vi "Create Default Attributes.vi"(5 "Unique ID":string, 7 "Process Executive Ref":refnum<data-value>, 11 "Wait in":refnum<class "Wait.lvclass">) -> (3 "Wait out":refnum<class "Wait.lvclass">)   [LabVIEW 2019, in "Wait.lvclass"]
uses:
  <vilib>/gpm_packages/@cs/Car-wash/Source/Process Steps/Wait/Wait.lvclass
  <vilib>/gpm_packages/@cs/test-executive/Source/Test Executive/ITestExecutive/ITest Executive.lvclass
  3f0b96d9-ec26-4894-9d74-60fba4d816d8.vi
  <vilib>/Utility/error.llb/Error Cluster From Error Code.vi
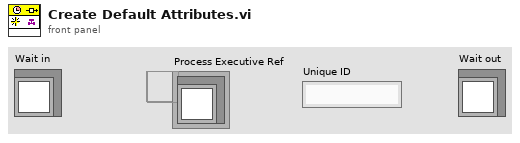
[diagram p1: front panel]
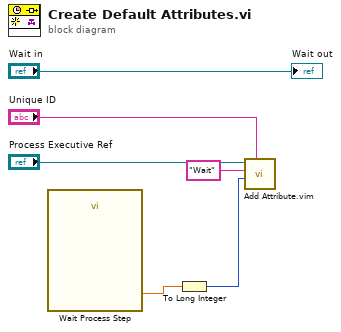
[diagram p0: block diagram]
diagram:
  n1 = call "Wait Process Step"() -> ("Wait Time"=w2:dbl)  [unwired: 17 in, 2 out]
  n2 = To Long Integer(number=w2) -> (32bit integer=w1:i32)
  n3 = call "Add Attribute.vim"("ID"="Unique ID", "Attribute"=w1, "Attribute Name"="Wait", "Test Executive Ref"="Process Executive Ref") -> ()  [unwired: 4 in, 4 out]
  "Wait out" <- "Wait in"
